vi "Add Noise and Delay.vi"(9 "delay iters":i32, 10 "Noise Mag":dbl, 11 "Numeric in":dbl[unit]) -> (3 "Numeric out":dbl[unit])   [LabVIEW 2020]
uses:
  dd44b683-bf39-4f0d-a5a3-5da23a0091c1.vi
  <vilib>/ptbypt/NI_PtbyPt.lvlib
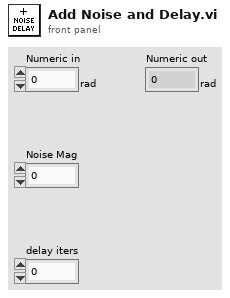
[diagram p1: front panel]
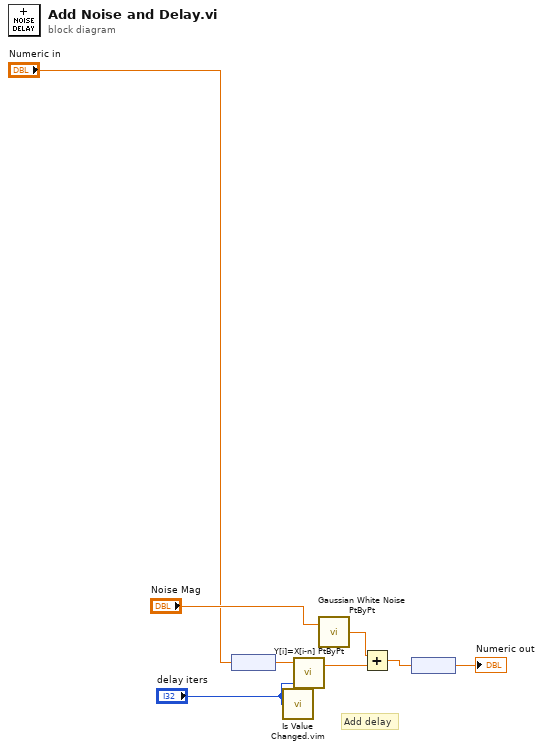
[diagram p0: block diagram]
diagram:
  # "Add delay"
  n1 = node("Numeric in") -> (w1:dbl)
  n2 = call "Is Value Changed.vim"("value"="delay iters") -> ("changed or first call?"=w3:bool)
  n3 = call <vilib>:"Y[i]=X[i-n] PtByPt.vi"("initialize"=w3, "shifts: n"="delay iters", "x"=w1) -> ("shifted x"=w7:dbl)  [unwired: 1 in, 1 out]
  n4 = call <vilib>:"Gaussian White Noise PtByPt.vi"("standard deviation"="Noise Mag") -> ("Gaussian white noise"=w9:dbl)  [unwired: 2 in]
  n5 = Add(x=w9, y=w7) -> (x+y=w6:dbl)
  n6 = node(w6) -> (→"Numeric out":dbl[unit])
